vi "9219 4Ch Universal Input.vi"(2 "9219 I/O":T4={"9219 Ch0"="NI 9219/CH0 Voltage", "9219 Ch1"="NI 9219/CH1 Temp", "9219 Ch2"="NI 9219/CH2 Resistance", "9219 Ch3"="NI 9219/CH3 Full Bridge", "9219 CJC"="NI 9219/CJC1"}, 3 "Voltage Range":T3 items=["+/- 60V", "+/- 15V", "+/- 4V", "+/- 1V", "+/- 125mV"], 4 "Resistance Range":T2 items=["10k", "1k"], 8 "Full Bridge Range":T1 items=["+/- 62.5mV/V", "+/- 7.8mV/V"]) -> (7 "Packets":u64[](array[numeric]))   [LabVIEW 2010]
uses:
  <vilib>/LabVIEW Targets/FPGA/cRIO/shared/nicrio_ModuleControls/nicrio_cRIO-9219_VoltageRange.ctl
  <vilib>/LabVIEW Targets/FPGA/cRIO/shared/nicrio_ModuleControls/nicrio_cRIO-9219_ResistanceRange.ctl
  <vilib>/LabVIEW Targets/FPGA/cRIO/shared/nicrio_ModuleControls/nicrio_cRIO-9219_FullBridgeRange.ctl
  <vilib>/eio/EIOPropertyNode/EIOPropertyNode.xnode
  <vilib>/rvi/eio/nirviEIOPropertyImplementation/nirviEIOPropertyImplementation.xnode
  <vilib>/eio/EIONode/EIONode.xnode
  <vilib>/rvi/eio/nirviEIOImplementation/nirviEIOImplementation.xnode
  <vilib>/rvi/eio/common/nirviEmuClasses.ctl
  <vilib>/rvi/eio/common/nirviEmuTemplatePropertySet_noerrors.vi
  <vilib>/rvi/eio/common/nirviEmuTemplateMethod_noerrors.vi
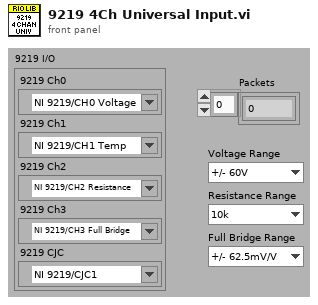
[diagram p1: front panel]
types:
  T1 = typedef "nicrio_cRIO-9219_FullBridgeRange.ctl" = u8
  T2 = typedef "nicrio_cRIO-9219_ResistanceRange.ctl" = u8
  T3 = typedef "nicrio_cRIO-9219_VoltageRange.ctl" = u8
  T4 = cluster{"9219 Ch0":refnum<k21>, "9219 Ch1":refnum<k21>, "9219 Ch2":refnum<k21>, "9219 Ch3":refnum<k21>, "9219 CJC":refnum<k21>}
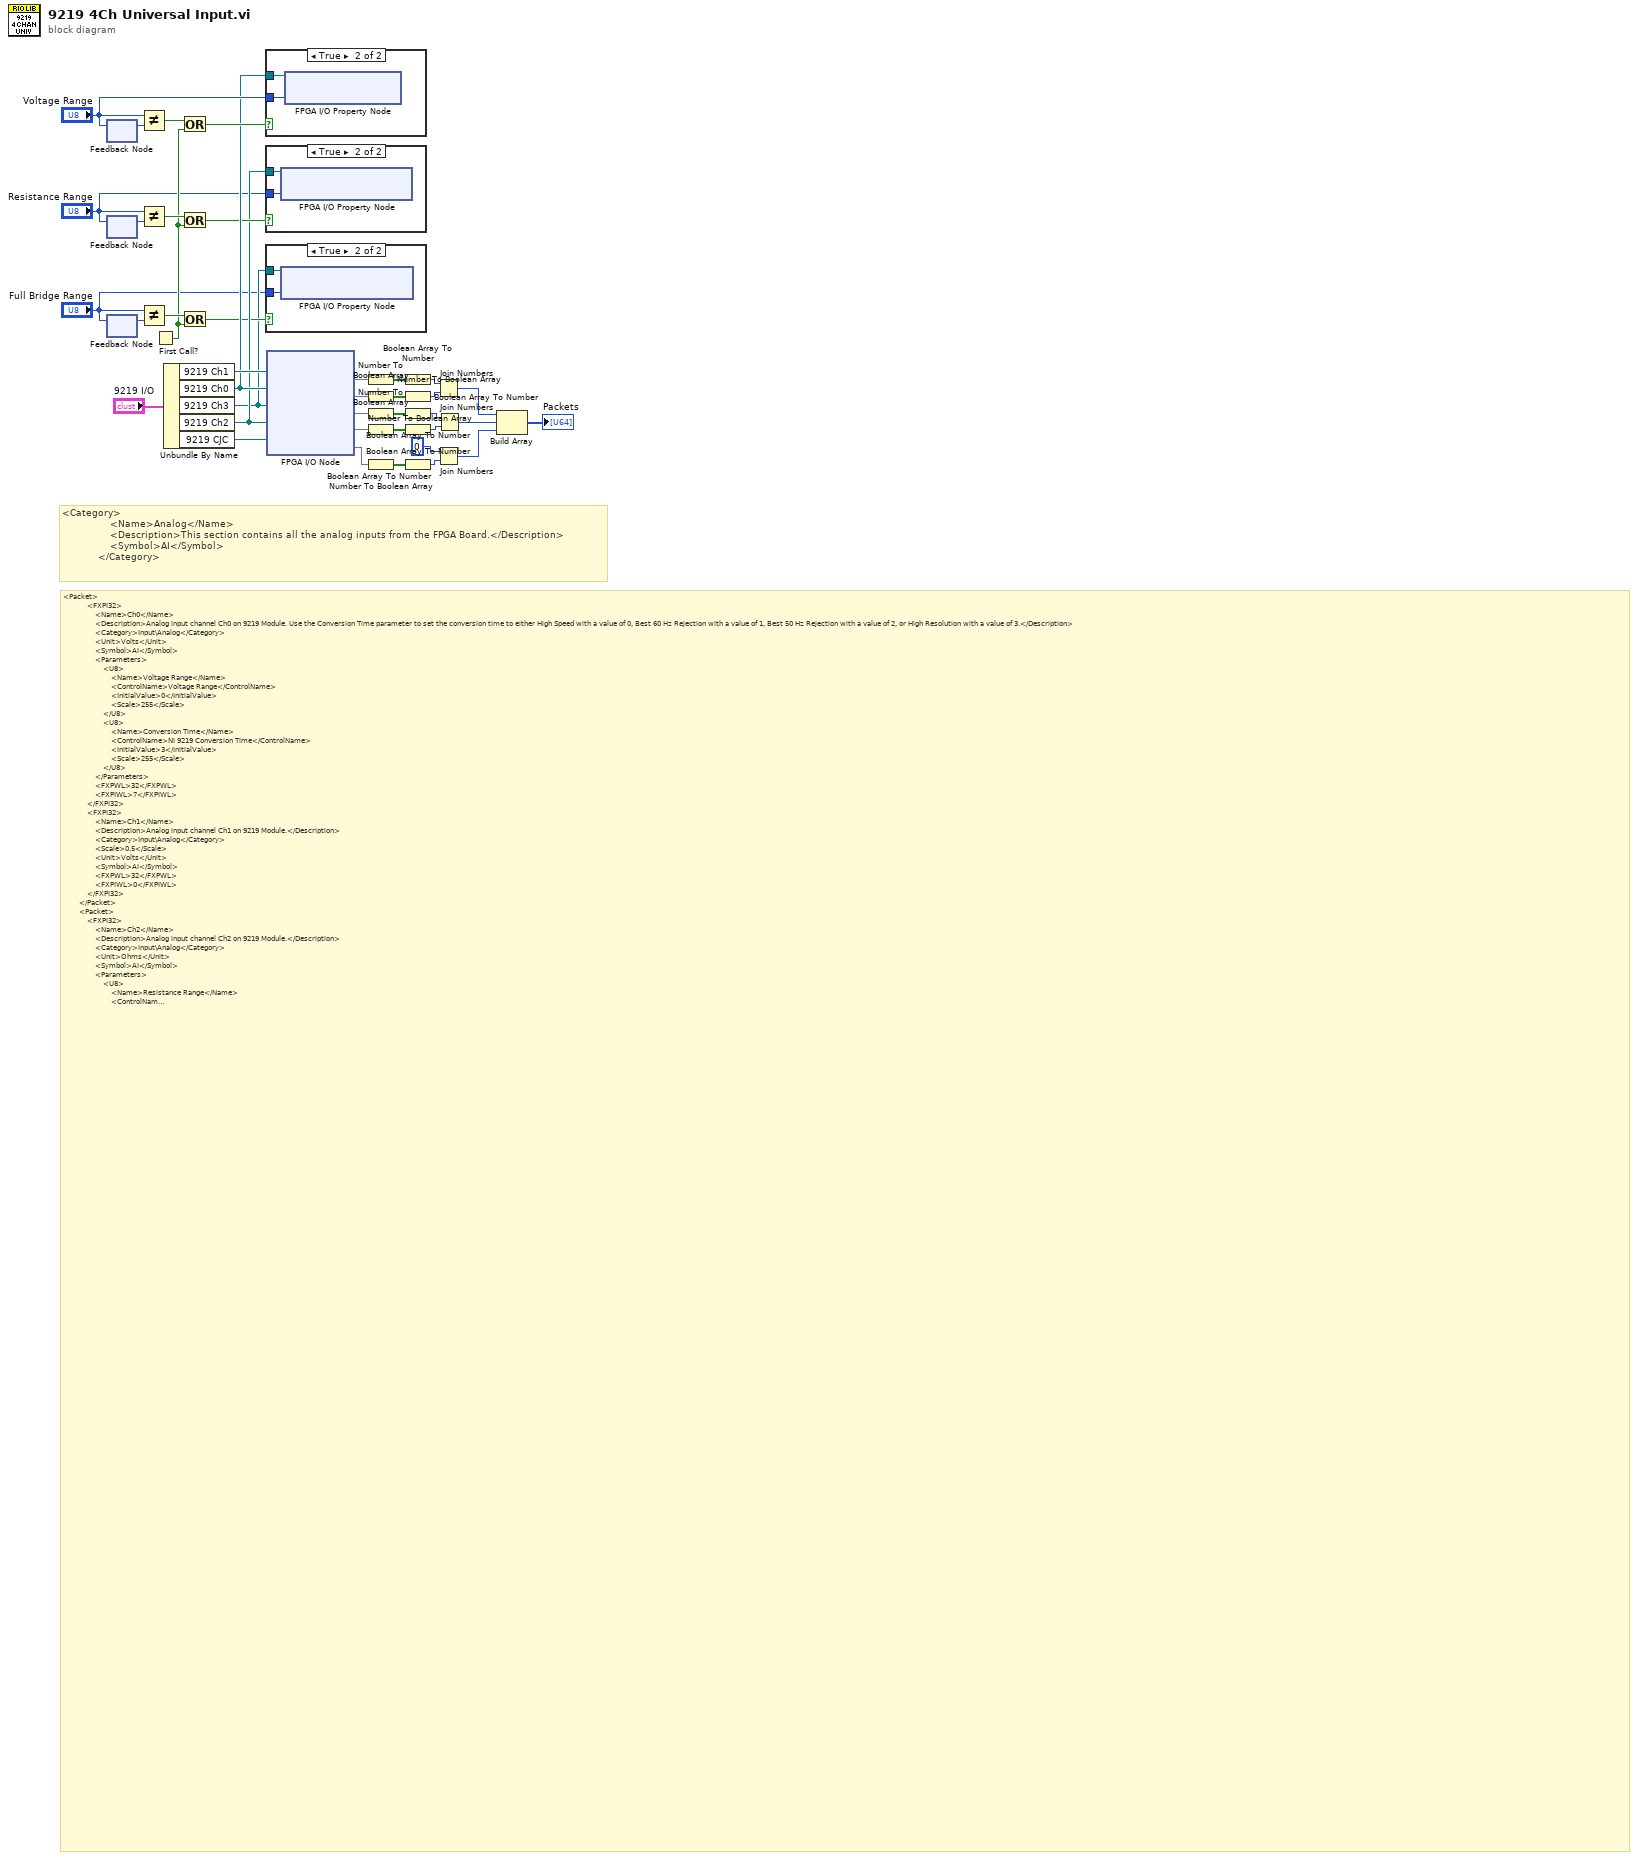
[diagram p0: block diagram]
diagram:
  # "<Category>\n                <Name>Analog</Name>\n                <Description>This section contains all the analog inputs from the FPGA Board.</Description>\n                <Symbol>AI</Symbol>\n            </Category>"
  # "<Packet>\n            <FXPI32>\n                <Name>Ch0</Name>\n                <Description>Analog input channel Ch0 on 9219 Module. Use the Conversion Time parameter to set the conversion time to either High Speed with a value of 0, Best 60 Hz Rejection with a value of 1, Best 50 Hz Rejection with a value of 2, or High Resolution with a value of 3.</Description>\n                <Category>Input\\Analog</Category>\n                <Unit>Volts</Unit>\n                <Symbol>AI</Symbol>\n                <Parameters>\n                    <U8>\n                        <Name>Voltage Range</Name>\n                        <ControlName>Voltage Range</ControlName>\n                        <InitialValue>0</InitialValue>\n                        <Scale>255</Scale>\n                    </U8>\n                    <U8>\n                        <Name>Conversion Time</Name>\n                        <ControlName>NI 9219 Conversion Time</ControlName>\n                        <InitialValue>3</InitialValue>\n                        <Scale>255</Scale>\n                    </U8>\n                </Parameters>\n                <FXPWL>32</FXPWL>\n                <FXPIWL>7</FXPIWL>\n            </FXPI32>\n            <FXPI32>\n                <Name>Ch1</Name>\n                <Description>Analog input channel Ch1 on 9219 Module.</Description>\n                <Category>Input\\Analog</Category>\n                <Scale>0.5</Scale>\n                <Unit>Volts</Unit>\n                <Symbol>AI</Symbol>\n                <FXPWL>32</FXPWL>\n                <FXPIWL>0</FXPIWL>\n            </FXPI32>\n        </Packet>\n        <Packet>\n            <FXPI32>\n                <Name>Ch2</Name>\n                <Description>Analog input channel Ch2 on 9219 Module.</Description>\n                <Category>Input\\Analog</Category>\n                <Unit>Ohms</Unit>\n                <Symbol>AI</Symbol>\n                <Parameters>\n                    <U8>\n                        <Name>Resistance Range</Name>\n                        <ControlName>Resistance Range</ControlName>\n                        <InitialValue>0</InitialValue>\n                        <Scale>255</Scale>\n                    </U8>\n                </Parameters>\n                <FXPWL>32</FXPWL>\n                <FXPIWL>14</FXPIWL>\n            </FXPI32>\n            <FXPI32>\n                <Name>Ch3</Name>\n                <Description>Analog input channel Ch3 on 9219 Module.</Description>\n                <Category>Input\\Analog</Category>\n                <Scale>0.5</Scale>\n                <Unit>V/V</Unit>\n                <Symbol>AI</Symbol>\n                <Parameters>\n                    <U8>\n                        <Name>Full Bridge Range</Name>\n                        <ControlName>Full Bridge Range</ControlName>\n                        <InitialValue>0</InitialValue>\n                        <Scale>255</Scale>\n                    </U8>\n                </Parameters>\n                <FXPWL>32</FXPWL>\n                <FXPIWL>0</FXPIWL>\n            </FXPI32>\n        </Packet>\n        <Packet>\n            <FXPI32>\n                <Name>CJC</Name>\n                <Description>Analog input channel CJC1 on 9219 Module.</Description>\n                <Category>Input\\Analog</Category>\n                <Scale>0.5</Scale>\n                <Unit>Volts</Unit>\n                <Symbol>AI</Symbol>\n                <FXPWL>32</FXPWL>\n                <FXPIWL>0</FXPIWL>\n            </FXPI32>\n        </Packet>"
  n1 = feedback-in #1("Voltage Range") -> ()
  n2 = feedback #1() -> (w15:T3)  [unwired: 1 in]
  n3 = feedback-in #2("Resistance Range") -> ()
  n4 = feedback #2() -> (w16:T2)  [unwired: 1 in]
  n5 = feedback-in #3("Full Bridge Range") -> ()
  n6 = feedback #3() -> (w17:T1)  [unwired: 1 in]
  n7 = Not Equal?(x="Voltage Range", y=w15) -> (x != y?=w14:bool)
  n8 = Not Equal?(x="Resistance Range", y=w16) -> (x != y?=w13:bool)
  n9 = Not Equal?(x="Full Bridge Range", y=w17) -> (x != y?=w12:bool)
  n10 = First Call?() -> (First Call?: T/F=w11:bool)
  n11 = Unbundle By Name("9219 I/O") -> ("9219 Ch1"=w8:refnum<k21>, "9219 Ch0"=w7:refnum<k21>, "9219 Ch3"=w2:refnum<k21>, "9219 Ch2"=w5:refnum<k21>, "9219 CJC"=w27:refnum<k21>)
  n12 = Or(x=w14, y=w11) -> (x .or. y?=w10:bool)
  n13 = Or(x=w13, y=w11) -> (x .or. y?=w6:bool)
  n14 = Or(x=w12, y=w11) -> (x .or. y?=w3:bool)
  n15 = case shown="True" w10 {
    tunnel: "Voltage Range" -> [_ w41]
    tunnel: w7 -> [_ w40]
    frame False {
    }
    frame True {
      n16 = xnode "FPGA I/O Property Node"("FPGA I/O In"=w40, "Voltage Range"=w41) -> ()  [unwired: 1 out]
    }
  }
  n17 = case shown="True" w6 {
    tunnel: "Resistance Range" -> [_ w50]
    tunnel: w5 -> [_ w49]
    frame False {
    }
    frame True {
      n18 = xnode "FPGA I/O Property Node"("FPGA I/O In"=w49, "Resistance Range"=w50) -> ()  [unwired: 1 out]
    }
  }
  n19 = case shown="True" w3 {
    tunnel: "Full Bridge Range" -> [_ w59]
    tunnel: w2 -> [_ w58]
    frame False {
    }
    frame True {
      n20 = xnode "FPGA I/O Property Node"("FPGA I/O In"=w58, "Full Bridge Range"=w59) -> ()  [unwired: 1 out]
    }
  }
  n21 = xnode "FPGA I/O Node"("FPGA I/O In"=w8, "FPGA I/O In"=w7, "FPGA I/O In"=w2, "FPGA I/O In"=w5, "FPGA I/O In"=w27) -> ("I/O Item"=w35:fxp<+/-,32,-1>, "I/O Item"=w36:fxp<+/-,32,7>, "I/O Item"=w24:fxp<+/-,32,-1>, "I/O Item"=w26:fxp<+,32,14>, "I/O Item"=w20:fxp<+/-,32,-1>)  [unwired: 5 out]
  n22 = Number To Boolean Array(number=w35) -> (Boolean array=w32:bool[])
  n23 = Number To Boolean Array(number=w36) -> (Boolean array=w33:bool[])
  n24 = Number To Boolean Array(number=w24) -> (Boolean array=w23:bool[])
  n25 = Number To Boolean Array(number=w26) -> (Boolean array=w34:bool[])
  n26 = Number To Boolean Array(number=w20) -> (Boolean array=w22:bool[])
  n27 = Boolean Array To Number(Boolean array=w32) -> (number=w37:u32)
  n28 = Boolean Array To Number(Boolean array=w33) -> (number=w38:u32)
  n29 = Boolean Array To Number(Boolean array=w23) -> (number=w25:u32)
  n30 = Boolean Array To Number(Boolean array=w34) -> (number=w39:u32)
  n31 = Boolean Array To Number(Boolean array=w22) -> (number=w21:u32)
  n32 = Join Numbers(hi=w37, lo=w38) -> ((hi.lo)=w30:u64)
  n33 = Join Numbers(hi=u32 0, lo=w21) -> ((hi.lo)=w19:u64)
  n34 = Join Numbers(hi=w25, lo=w39) -> ((hi.lo)=w31:u64)
  n35 = Build Array(w30, w31, w19) -> (→"Packets":u64[])
